vi "Initialization VI.vi"(8 "error in (no error)":errorcluster, 10 "Custom XML":string, 11 "Device Item Ref in":T1 format="%.0x") -> (0 "error out":errorcluster, 3 "Device Item Ref out":T1 format="%.0x")   [LabVIEW 2020, in "G5 Regatron Custom Device System Explorer.lvlib"]
uses:
  G5 Regatron Custom Device System Explorer.lvlib
  <vilib>/NI VeriStand/Custom Device API/Custom Device Item Ref.ctl
  <vilib>/NI VeriStand/Custom Device API/Custom Device Channel.ctl
  <vilib>/NI VeriStand/Custom Device API/Custom Device Channel Type.ctl
  <vilib>/NI/NI VeriStand Custom Device Import and Export Tool/ImportExport.lvlib
  <vilib>/NI VeriStand/Custom Device API/Custom Device API.lvlib
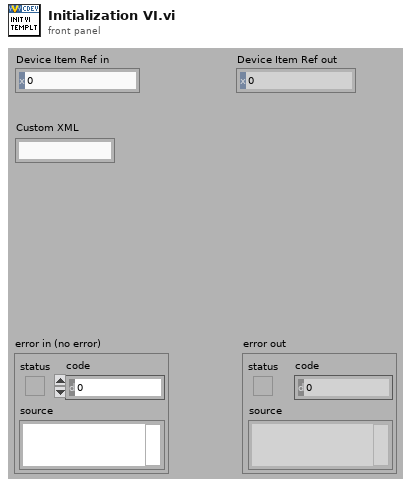
[diagram p1: front panel]
types:
  T1 = typedef "Custom Device API.lvlib/Custom Device Item Ref.ctl" = u64
  T2 = typedef "Custom Device API.lvlib/Custom Device Channel.ctl" = cluster{"Type":T3, "Units":string, "Default Value":dbl, "Faultable":bool, "Scalable":bool}
  T3 = typedef "Custom Device API.lvlib/Custom Device Channel Type.ctl" = enum16{"Input", "Output"}
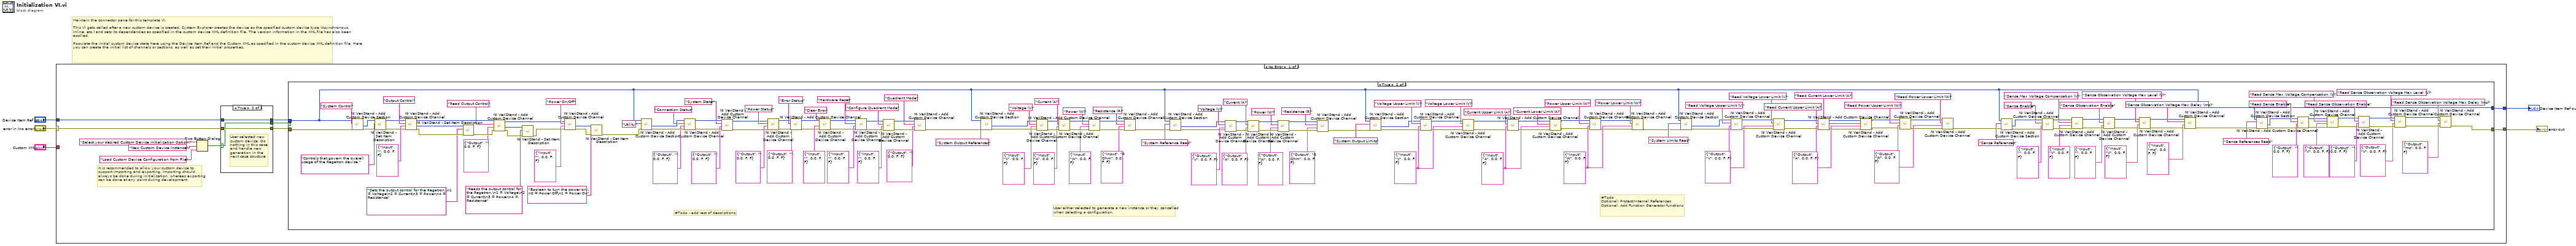
[diagram p0: block diagram]
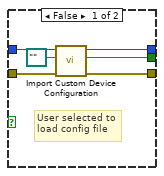
[diagram p3: hidden frame]
diagram:
  # "Maintain the connector pane for this template VI.\n\nThis VI gets called after a new custom device is created. System Explorer creates the device as the specified custom device type (Asynchronous, Inline, etc.) and sets its dependencies as specified in the custom device XML definition file. The version information in the XML file has also been applied.\n\nPopulate the initial custom device state here using the Device Item Ref and the Custom XML as specified in the custom device XML definition file. Here you can create the initial list of channels or sections, as well as set their initial properties."
  n1 = case shown="No Error" "error in (no error)" {
    selector: "error in (no error)" -> [w11 w217]
    tunnel: [w6 w217] -> w5
    tunnel: [w7 w216] -> w3
    tunnel: "Device Item Ref in" -> [w12 w216]
    tunnel: "Custom XML" -> [_ _]
    frame No Error {
      # "It is recommended to allow your custom device to\nsupport importing and exporting. Importing should\nalways be done during initialization, whereas exporting\ncan be done at any point during development"
      n2 = Two Button Dialog(message="Select your desired Custom Device Initialization Option:", 1:"Load Custom Device Configuration from File" ("F button name (\"Cancel\")"), 2:"New Custom Device Instance" ("T button name (\"OK\")")) -> (T button?=w13:bool)
      n3 = case shown="True" w13 {
        selector: w13 -> [_ w213]
        tunnel: w12 -> [w212 w215]
        tunnel: [w211 w215] -> w8
        tunnel: w11 -> [w209 w214]
        tunnel: [w208 w214] -> w10
        tunnel: [w207 w213] -> w9
        frame False {
          # "User selected to\nload config file"
          n4 = call <vilib>:"Import Custom Device Configuration.vi"("error in (no error)"=w209, "Path"=path "", "NodeID"=w212) -> ("error out"=w208:errorcluster, "cancelled"=w207:bool, "NodeID out"=w211:u64)  [unwired: 6 in]
        }
        frame True {
          # "User selected new\ncustom device. Do\nnothing in this case\nand handle new\ngeneration in the\nnext case structure"
        }
      }
      n5 = case shown="True" w9 {
        tunnel: w8 -> [w18 w28]
        tunnel: w10 -> [w17 w182]
        tunnel: [w17 w29] -> w6
        tunnel: [w18 w28] -> w7
        frame False {
          # "User selected to import from configuration and didn't cancel import"
        }
        frame True {
          w60 = T2 {"Type"=enum."Output", "Units"="W", "Default Value"=0.0, "Faultable"=FALSE, "Scalable"=FALSE} ("Channel")
          w65 = T2 {"Type"=enum."Output", "Units"="V", "Default Value"=0.0, "Faultable"=FALSE, "Scalable"=FALSE} ("Channel")
          w71 = T2 {"Type"=enum."Output", "Units"="A", "Default Value"=0.0, "Faultable"=FALSE, "Scalable"=FALSE} ("Channel")
          w134 = T2 {"Type"=enum."Input", "Units"="W", "Default Value"=0.0, "Faultable"=FALSE, "Scalable"=FALSE} ("Channel")
          w139 = T2 {"Type"=enum."Input", "Units"="V", "Default Value"=0.0, "Faultable"=FALSE, "Scalable"=FALSE} ("Channel")
          w193 = T2 {"Type"=enum."Input", "Units"="A", "Default Value"=0.0, "Faultable"=FALSE, "Scalable"=FALSE} ("Channel")
          # "#Todo - add rest of descriptions."
          # "#Todo\nOptional: Protect/Internal References\nOptional: Add Function Generator functions"
          # "User either selected to generate a new instance or they cancelled\nwhen selecting a configuration."
          n6 = call <vilib>:"NI VeriStand - Add Custom Device Section.vi"("error in (no error)"=w182, "Section Name"="System Control", "Parent Ref in"=w28) -> ("error out"=w121:errorcluster, "Section Ptr"=w119:T1)  [unwired: 5 in, 2 out]
          n7 = call <vilib>:"NI VeriStand - Set Item Description.vi"("error in (no error)"=w121, "Description"="Controls that govern the overall usage of the Regatron device.", "Item Ref in"=w119) -> ("error out"=w120:errorcluster, "Item Ref out"=w118:T1)  [unwired: 6 in, 1 out]
          n8 = call <vilib>:"NI VeriStand - Add Custom Device Channel.vi"("error in (no error)"=w120, "Channel"=T2 {"Type"=enum."Input", "Units"="", "Default Value"=0.0, "Faultable"=FALSE, "Scalable"=FALSE}, "Channel Name"="Output Control", "Parent Ref in"=w118) -> ("error out"=w126:errorcluster, "Channel Ref"=w127:T1, "Parent Ref out"=w27:T1)  [unwired: 4 in, 1 out]
          n9 = call <vilib>:"NI VeriStand - Set Item Description.vi"("error in (no error)"=w126, "Description"="Sets the output control for the Regatron.\n1 = Voltage\n2 = Current\n3 = Power\n4 = Resistance", "Item Ref in"=w127) -> ("error out"=w25:errorcluster)  [unwired: 6 in, 2 out]
          n10 = call <vilib>:"NI VeriStand - Add Custom Device Channel.vi"("error in (no error)"=w25, "Channel"=T2 {"Type"=enum."Output", "Units"="", "Default Value"=0.0, "Faultable"=FALSE, "Scalable"=FALSE}, "Channel Name"="Read Output Control", "Parent Ref in"=w27) -> ("error out"=w22:errorcluster, "Channel Ref"=w23:T1, "Parent Ref out"=w26:T1)  [unwired: 4 in, 1 out]
          n11 = call <vilib>:"NI VeriStand - Set Item Description.vi"("error in (no error)"=w22, "Description"="Reads the output control for the Regatron.\n1 = Voltage\n2 = Current\n3 = Power\n4 = Resistance", "Item Ref in"=w23) -> ("error out"=w21:errorcluster)  [unwired: 6 in, 2 out]
          n12 = call <vilib>:"NI VeriStand - Add Custom Device Channel.vi"("error in (no error)"=w21, "Channel"=T2 {"Type"=enum."Input", "Units"="", "Default Value"=0.0, "Faultable"=FALSE, "Scalable"=FALSE}, "Channel Name"="Power On/Off", "Parent Ref in"=w26) -> ("error out"=w124:errorcluster, "Channel Ref"=w123:T1)  [unwired: 4 in, 2 out]
          n13 = call <vilib>:"NI VeriStand - Set Item Description.vi"("error in (no error)"=w124, "Description"="Boolean to turn the power on.\n0 = Power Off\n1 = Power On", "Item Ref in"=w123) -> ("error out"=w116:errorcluster)  [unwired: 6 in, 2 out]
          n14 = call <vilib>:"NI VeriStand - Add Custom Device Section.vi"("error in (no error)"=w116, "Section Name"="Utility", "Parent Ref in"=w28) -> ("error out"=w172:errorcluster, "Section Ptr"=w170:T1)  [unwired: 5 in, 2 out]
          n15 = call <vilib>:"NI VeriStand - Add Custom Device Channel.vi"("error in (no error)"=w172, "Channel"=T2 {"Type"=enum."Output", "Units"="", "Default Value"=0.0, "Faultable"=FALSE, "Scalable"=FALSE}, "Channel Name"="Connection Status", "Parent Ref in"=w170) -> ("error out"=w113:errorcluster, "Parent Ref out"=w115:T1)  [unwired: 4 in, 2 out]
          n16 = call <vilib>:"NI VeriStand - Add Custom Device Channel.vi"("error in (no error)"=w113, "Channel"=T2 {"Type"=enum."Output", "Units"="", "Default Value"=0.0, "Faultable"=FALSE, "Scalable"=FALSE}, "Channel Name"="System State", "Parent Ref in"=w115) -> ("error out"=w112:errorcluster, "Parent Ref out"=w114:T1)  [unwired: 4 in, 2 out]
          n17 = call <vilib>:"NI VeriStand - Add Custom Device Channel.vi"("error in (no error)"=w112, "Channel"=T2 {"Type"=enum."Output", "Units"="", "Default Value"=0.0, "Faultable"=FALSE, "Scalable"=FALSE}, "Channel Name"="Power Status", "Parent Ref in"=w114) -> ("error out"=w178:errorcluster, "Parent Ref out"=w180:T1)  [unwired: 4 in, 2 out]
          n18 = call <vilib>:"NI VeriStand - Add Custom Device Channel.vi"("error in (no error)"=w178, "Channel"=T2 {"Type"=enum."Output", "Units"="", "Default Value"=0.0, "Faultable"=FALSE, "Scalable"=FALSE}, "Channel Name"="Error Status", "Parent Ref in"=w180) -> ("error out"=w177:errorcluster, "Parent Ref out"=w179:T1)  [unwired: 4 in, 2 out]
          n19 = call <vilib>:"NI VeriStand - Add Custom Device Channel.vi"("error in (no error)"=w177, "Channel"=T2 {"Type"=enum."Input", "Units"="", "Default Value"=0.0, "Faultable"=FALSE, "Scalable"=FALSE}, "Channel Name"="Clear Error", "Parent Ref in"=w179) -> ("error out"=w88:errorcluster, "Parent Ref out"=w87:T1)  [unwired: 4 in, 2 out]
          n20 = call <vilib>:"NI VeriStand - Add Custom Device Channel.vi"("error in (no error)"=w88, "Channel"=T2 {"Type"=enum."Input", "Units"="", "Default Value"=0.0, "Faultable"=FALSE, "Scalable"=FALSE}, "Channel Name"="Hardware Reset", "Parent Ref in"=w87) -> ("error out"=w83:errorcluster, "Parent Ref out"=w84:T1)  [unwired: 4 in, 2 out]
          n21 = call <vilib>:"NI VeriStand - Add Custom Device Channel.vi"("error in (no error)"=w83, "Channel"=T2 {"Type"=enum."Input", "Units"="", "Default Value"=0.0, "Faultable"=FALSE, "Scalable"=FALSE}, "Channel Name"="Configure Quadrant Mode", "Parent Ref in"=w84) -> ("error out"=w80:errorcluster, "Parent Ref out"=w79:T1)  [unwired: 4 in, 2 out]
          n22 = call <vilib>:"NI VeriStand - Add Custom Device Channel.vi"("error in (no error)"=w80, "Channel"=T2 {"Type"=enum."Output", "Units"="", "Default Value"=0.0, "Faultable"=FALSE, "Scalable"=FALSE}, "Channel Name"="Quadrant Mode", "Parent Ref in"=w79) -> ("error out"=w76:errorcluster)  [unwired: 4 in, 3 out]
          n23 = call <vilib>:"NI VeriStand - Add Custom Device Section.vi"("error in (no error)"=w76, "Section Name"="System Output References", "Parent Ref in"=w28) -> ("error out"=w174:errorcluster, "Section Ptr"=w175:T1)  [unwired: 5 in, 2 out]
          n24 = call <vilib>:"NI VeriStand - Add Custom Device Channel.vi"("error in (no error)"=w174, "Channel"=T2 {"Type"=enum."Input", "Units"="V", "Default Value"=0.0, "Faultable"=FALSE, "Scalable"=FALSE}, "Channel Name"="Voltage (V)", "Parent Ref in"=w175) -> ("error out"=w204:errorcluster, "Parent Ref out"=w203:T1)  [unwired: 4 in, 2 out]
          n25 = call <vilib>:"NI VeriStand - Add Custom Device Channel.vi"("error in (no error)"=w204, "Channel"=T2 {"Type"=enum."Input", "Units"="A", "Default Value"=0.0, "Faultable"=FALSE, "Scalable"=FALSE}, "Channel Name"="Current (A)", "Parent Ref in"=w203) -> ("error out"=w202:errorcluster, "Parent Ref out"=w201:T1)  [unwired: 4 in, 2 out]
          n26 = call <vilib>:"NI VeriStand - Add Custom Device Channel.vi"("error in (no error)"=w202, "Channel"=T2 {"Type"=enum."Input", "Units"="W", "Default Value"=0.0, "Faultable"=FALSE, "Scalable"=FALSE}, "Channel Name"="Power (W)", "Parent Ref in"=w201) -> ("error out"=w199:errorcluster, "Parent Ref out"=w198:T1)  [unwired: 4 in, 2 out]
          n27 = call <vilib>:"NI VeriStand - Add Custom Device Channel.vi"("error in (no error)"=w199, "Channel"=T2 {"Type"=enum."Input", "Units"="R Ohm", "Default Value"=0.0, "Faultable"=FALSE, "Scalable"=FALSE}, "Channel Name"="Resistance (R)", "Parent Ref in"=w198) -> ("error out"=w145:errorcluster)  [unwired: 4 in, 3 out]
          n28 = call <vilib>:"NI VeriStand - Add Custom Device Section.vi"("error in (no error)"=w145, "Section Name"="System Reference Read", "Parent Ref in"=w28) -> ("error out"=w151:errorcluster, "Section Ptr"=w152:T1)  [unwired: 5 in, 2 out]
          n29 = call <vilib>:"NI VeriStand - Add Custom Device Channel.vi"("error in (no error)"=w151, "Channel"=T2 {"Type"=enum."Output", "Units"="V", "Default Value"=0.0, "Faultable"=FALSE, "Scalable"=FALSE}, "Channel Name"="Voltage (V)", "Parent Ref in"=w152) -> ("error out"=w160:errorcluster, "Parent Ref out"=w159:T1)  [unwired: 4 in, 2 out]
          n30 = call <vilib>:"NI VeriStand - Add Custom Device Channel.vi"("error in (no error)"=w160, "Channel"=T2 {"Type"=enum."Output", "Units"="A", "Default Value"=0.0, "Faultable"=FALSE, "Scalable"=FALSE}, "Channel Name"="Current (A)", "Parent Ref in"=w159) -> ("error out"=w158:errorcluster, "Parent Ref out"=w157:T1)  [unwired: 4 in, 2 out]
          n31 = call <vilib>:"NI VeriStand - Add Custom Device Channel.vi"("error in (no error)"=w158, "Channel"=T2 {"Type"=enum."Output", "Units"="W", "Default Value"=0.0, "Faultable"=FALSE, "Scalable"=FALSE}, "Channel Name"="Power (W)", "Parent Ref in"=w157) -> ("error out"=w155:errorcluster, "Parent Ref out"=w154:T1)  [unwired: 4 in, 2 out]
          n32 = call <vilib>:"NI VeriStand - Add Custom Device Channel.vi"("error in (no error)"=w155, "Channel"=T2 {"Type"=enum."Output", "Units"="R Ohm", "Default Value"=0.0, "Faultable"=FALSE, "Scalable"=FALSE}, "Channel Name"="Resistance (R)", "Parent Ref in"=w154) -> ("error out"=w144:errorcluster)  [unwired: 4 in, 3 out]
          n33 = call <vilib>:"NI VeriStand - Add Custom Device Section.vi"("error in (no error)"=w144, "Section Name"="System Output Limits", "Parent Ref in"=w28) -> ("error out"=w138:errorcluster, "Section Ptr"=w137:T1)  [unwired: 5 in, 2 out]
          n34 = call <vilib>:"NI VeriStand - Add Custom Device Channel.vi"("error in (no error)"=w138, "Channel"=w139, "Channel Name"="Voltage Upper Limit (V)", "Parent Ref in"=w137) -> ("error out"=w142:errorcluster, "Parent Ref out"=w141:T1)  [unwired: 4 in, 2 out]
          n35 = call <vilib>:"NI VeriStand - Add Custom Device Channel.vi"("error in (no error)"=w142, "Channel"=w139, "Channel Name"="Voltage Lower Limit (V)", "Parent Ref in"=w141) -> ("error out"=w135:errorcluster, "Parent Ref out"=w136:T1)  [unwired: 4 in, 2 out]
          n36 = call <vilib>:"NI VeriStand - Add Custom Device Channel.vi"("error in (no error)"=w135, "Channel"=w193, "Channel Name"="Current Upper Limit (A)", "Parent Ref in"=w136) -> ("error out"=w196:errorcluster, "Parent Ref out"=w195:T1)  [unwired: 4 in, 2 out]
          n37 = call <vilib>:"NI VeriStand - Add Custom Device Channel.vi"("error in (no error)"=w196, "Channel"=w193, "Channel Name"="Current Lower Limit (A)", "Parent Ref in"=w195) -> ("error out"=w128:errorcluster, "Parent Ref out"=w129:T1)  [unwired: 4 in, 2 out]
          n38 = call <vilib>:"NI VeriStand - Add Custom Device Channel.vi"("error in (no error)"=w128, "Channel"=w134, "Channel Name"="Power Upper Limit (W)", "Parent Ref in"=w129) -> ("error out"=w131:errorcluster, "Parent Ref out"=w132:T1)  [unwired: 4 in, 2 out]
          n39 = call <vilib>:"NI VeriStand - Add Custom Device Channel.vi"("error in (no error)"=w131, "Channel"=w134, "Channel Name"="Power Lower Limit (W)", "Parent Ref in"=w132) -> ("error out"=w53:errorcluster)  [unwired: 4 in, 3 out]
          n40 = call <vilib>:"NI VeriStand - Add Custom Device Section.vi"("error in (no error)"=w53, "Section Name"="System Limits Read", "Parent Ref in"=w28) -> ("error out"=w64:errorcluster, "Section Ptr"=w63:T1)  [unwired: 5 in, 2 out]
          n41 = call <vilib>:"NI VeriStand - Add Custom Device Channel.vi"("error in (no error)"=w64, "Channel"=w65, "Channel Name"="Read Voltage Upper Limit (V)", "Parent Ref in"=w63) -> ("error out"=w68:errorcluster, "Parent Ref out"=w67:T1)  [unwired: 4 in, 2 out]
          n42 = call <vilib>:"NI VeriStand - Add Custom Device Channel.vi"("error in (no error)"=w68, "Channel"=w65, "Channel Name"="Read Voltage Lower Limit (V)", "Parent Ref in"=w67) -> ("error out"=w61:errorcluster, "Parent Ref out"=w62:T1)  [unwired: 4 in, 2 out]
          n43 = call <vilib>:"NI VeriStand - Add Custom Device Channel.vi"("error in (no error)"=w61, "Channel"=w71, "Channel Name"="Read Current Upper Limit (A)", "Parent Ref in"=w62) -> ("error out"=w74:errorcluster, "Parent Ref out"=w73:T1)  [unwired: 4 in, 2 out]
          n44 = call <vilib>:"NI VeriStand - Add Custom Device Channel.vi"("error in (no error)"=w74, "Channel"=w71, "Channel Name"="Read Current Lower Limit (A)", "Parent Ref in"=w73) -> ("error out"=w54:errorcluster, "Parent Ref out"=w55:T1)  [unwired: 4 in, 2 out]
          n45 = call <vilib>:"NI VeriStand - Add Custom Device Channel.vi"("error in (no error)"=w54, "Channel"=w60, "Channel Name"="Read Power Upper Limit (W)", "Parent Ref in"=w55) -> ("error out"=w57:errorcluster, "Parent Ref out"=w58:T1)  [unwired: 4 in, 2 out]
          n46 = call <vilib>:"NI VeriStand - Add Custom Device Channel.vi"("error in (no error)"=w57, "Channel"=w60, "Channel Name"="Read Power Lower Limit (W)", "Parent Ref in"=w58) -> ("error out"=w52:errorcluster)  [unwired: 4 in, 3 out]
          n47 = call <vilib>:"NI VeriStand - Add Custom Device Section.vi"("error in (no error)"=w52, "Section Name"="Sense References", "Parent Ref in"=w28) -> ("error out"=w108:errorcluster, "Section Ptr"=w107:T1)  [unwired: 5 in, 2 out]
          n48 = call <vilib>:"NI VeriStand - Add Custom Device Channel.vi"("error in (no error)"=w108, "Channel"=T2 {"Type"=enum."Input", "Units"="", "Default Value"=0.0, "Faultable"=FALSE, "Scalable"=FALSE}, "Channel Name"="Sense Enable", "Parent Ref in"=w107) -> ("error out"=w104:errorcluster, "Parent Ref out"=w103:T1)  [unwired: 4 in, 2 out]
          n49 = call <vilib>:"NI VeriStand - Add Custom Device Channel.vi"("error in (no error)"=w104, "Channel"=T2 {"Type"=enum."Input", "Units"="V", "Default Value"=0.0, "Faultable"=FALSE, "Scalable"=FALSE}, "Channel Name"="Sense Max Voltage Compensation (V)", "Parent Ref in"=w103) -> ("error out"=w100:errorcluster, "Parent Ref out"=w99:T1)  [unwired: 4 in, 2 out]
          n50 = call <vilib>:"NI VeriStand - Add Custom Device Channel.vi"("error in (no error)"=w100, "Channel"=T2 {"Type"=enum."Input", "Units"="", "Default Value"=0.0, "Faultable"=FALSE, "Scalable"=FALSE}, "Channel Name"="Sense Observation Enable", "Parent Ref in"=w99) -> ("error out"=w91:errorcluster, "Parent Ref out"=w92:T1)  [unwired: 4 in, 2 out]
          n51 = call <vilib>:"NI VeriStand - Add Custom Device Channel.vi"("error in (no error)"=w91, "Channel"=T2 {"Type"=enum."Input", "Units"="V", "Default Value"=0.0, "Faultable"=FALSE, "Scalable"=FALSE}, "Channel Name"="Sense Observation Voltage Max Level (V)", "Parent Ref in"=w92) -> ("error out"=w89:errorcluster, "Parent Ref out"=w90:T1)  [unwired: 4 in, 2 out]
          n52 = call <vilib>:"NI VeriStand - Add Custom Device Channel.vi"("error in (no error)"=w89, "Channel"=T2 {"Type"=enum."Input", "Units"="ms", "Default Value"=0.0, "Faultable"=FALSE, "Scalable"=FALSE}, "Channel Name"="Sense Observation Voltage Max Delay (ms)", "Parent Ref in"=w90) -> ("error out"=w30:errorcluster)  [unwired: 4 in, 3 out]
          n53 = call <vilib>:"NI VeriStand - Add Custom Device Section.vi"("error in (no error)"=w30, "Section Name"="Sense References Read", "Parent Ref in"=w28) -> ("error out"=w32:errorcluster, "Section Ptr"=w33:T1)  [unwired: 5 in, 2 out]
          n54 = call <vilib>:"NI VeriStand - Add Custom Device Channel.vi"("error in (no error)"=w32, "Channel"=T2 {"Type"=enum."Output", "Units"="", "Default Value"=0.0, "Faultable"=FALSE, "Scalable"=FALSE}, "Channel Name"="Read Sense Enable", "Parent Ref in"=w33) -> ("error out"=w36:errorcluster, "Parent Ref out"=w37:T1)  [unwired: 4 in, 2 out]
          n55 = call <vilib>:"NI VeriStand - Add Custom Device Channel.vi"("error in (no error)"=w36, "Channel"=T2 {"Type"=enum."Output", "Units"="V", "Default Value"=0.0, "Faultable"=FALSE, "Scalable"=FALSE}, "Channel Name"="Read Sense Max Voltage Compensation (V)", "Parent Ref in"=w37) -> ("error out"=w40:errorcluster, "Parent Ref out"=w41:T1)  [unwired: 4 in, 2 out]
          n56 = call <vilib>:"NI VeriStand - Add Custom Device Channel.vi"("error in (no error)"=w40, "Channel"=T2 {"Type"=enum."Output", "Units"="", "Default Value"=0.0, "Faultable"=FALSE, "Scalable"=FALSE}, "Channel Name"="Read Sense Observation Enable", "Parent Ref in"=w41) -> ("error out"=w49:errorcluster, "Parent Ref out"=w48:T1)  [unwired: 4 in, 2 out]
          n57 = call <vilib>:"NI VeriStand - Add Custom Device Channel.vi"("error in (no error)"=w49, "Channel"=T2 {"Type"=enum."Output", "Units"="V", "Default Value"=0.0, "Faultable"=FALSE, "Scalable"=FALSE}, "Channel Name"="Read Sense Observation Voltage Max Level (V)", "Parent Ref in"=w48) -> ("error out"=w51:errorcluster, "Parent Ref out"=w50:T1)  [unwired: 4 in, 2 out]
          n58 = call <vilib>:"NI VeriStand - Add Custom Device Channel.vi"("error in (no error)"=w51, "Channel"=T2 {"Type"=enum."Output", "Units"="ms", "Default Value"=0.0, "Faultable"=FALSE, "Scalable"=FALSE}, "Channel Name"="Read Sense Observation Voltage Max Delay (ms)", "Parent Ref in"=w50) -> ("error out"=w29:errorcluster)  [unwired: 4 in, 3 out]
        }
      }
    }
    frame Error {
    }
  }
  "error out" <- w5
  "Device Item Ref out" <- w3
